vi "Write Display Control.vi"(8 "error in (no error)":errorcluster, 9 "Display Control":T1, 10 "Session In":refnum<class "Session.lvclass">, 11 "Grove I2C LCD in":refnum<class "Grove I2C LCD.lvclass">) -> (0 "error out":errorcluster, 2 "Session Out":refnum<class "Session.lvclass">, 3 "Grove I2C LCD out":refnum<class "Grove I2C LCD.lvclass">)   [LabVIEW 2020, in "CTI-Peripheral.lvlib" / "Grove I2C LCD.lvclass"]
uses:
  Grove I2C LCD.lvclass
  HD44780 LCD/Display Control.ctl
  CTI/Session/Session.lvclass
  HD44780 LCD/Command.ctl
  Grove I2C LCD.lvclass/Grove I2C LCD.ctl
  HD44780 LCD/HD44780 LCD.lvlib
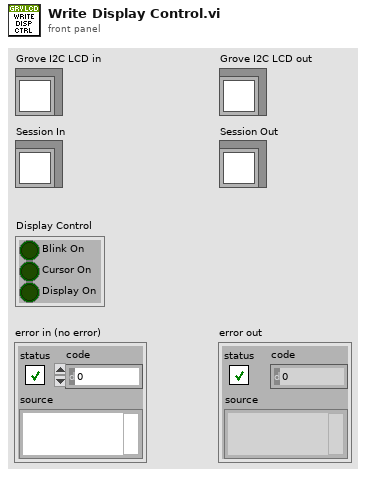
[diagram p1: front panel]
types:
  T1 = typedef "CTI-Peripheral.lvlib/HD44780 LCD.lvlib/Display Control.ctl" = cluster{"Blink On":bool, "Cursor On":bool, "Display On":bool}
  T2 = typedef "CTI-Peripheral.lvlib/HD44780 LCD.lvlib/Command.ctl" = enum16{"ClearDisplay", "ReturnHome", "EntryModeSet", "DisplayControl", "CursorShift", "FunctionSet", "SetCGRamAddr", "SetDDRamAddr"}
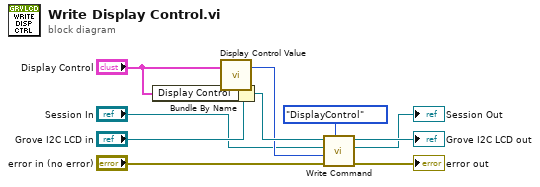
[diagram p0: block diagram]
diagram:
  n1 = Bundle By Name(cluster="Grove I2C LCD in", "Display Control"="Display Control") -> (w6:refnum<class "Grove I2C LCD.lvclass">)
  n2 = call "Display Control Value.vi"("Display Control"="Display Control") -> ("DCtrl Value"=w3:u8)  [unwired: 6 in]
  n3 = call "Write Command.vi"("Command"=Command."DisplayControl", "error in (no error)"="error in (no error)", "Value"=w3, "Session In"="Session In", "Grove I2C LCD in"=w6) -> ("error out"=→"error out":errorcluster, "Session Out"=→"Session Out":refnum<class "Session.lvclass">, "Grove I2C LCD out"=→"Grove I2C LCD out":refnum<class "Grove I2C LCD.lvclass">)  [unwired: 4 in]
